vi "STD校准信息读取.vi"(8 "Error in":errorcluster caption="Error in (no error)", 11 "Slave ID":u8=1) -> (0 "error out":errorcluster, 2 "结果字符串":string, 3 "校准信息读取":T1 {"校准类型" items=["单点校准"=1, "两点校准"=2, "三点校准"=3]})   [LabVIEW 2016, in "斯坦道原位多参数.lvlib"]
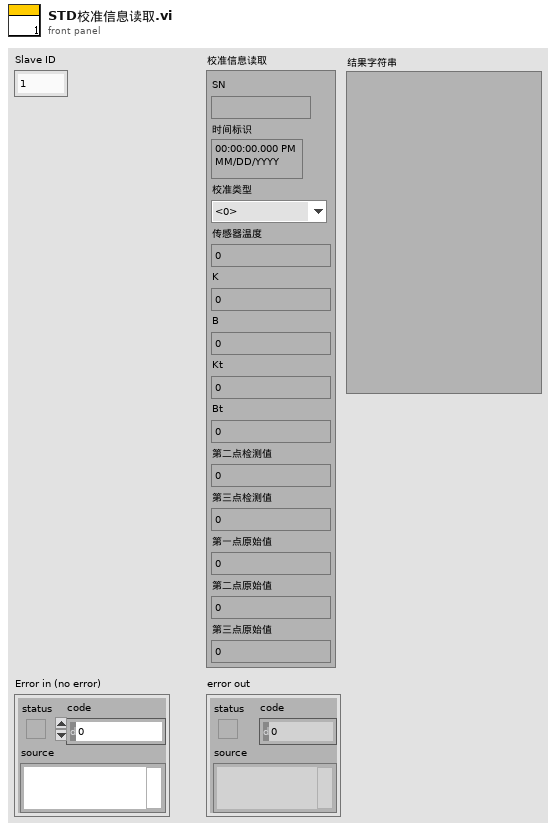
[diagram p1: front panel]
types:
  T1 = cluster{"SN":string, "时间标识":timestamp, "校准类型":u16, "传感器温度":sgl, "K":sgl, "B":sgl, "Kt":sgl, "Bt":sgl, "第二点检测值":sgl, "第三点检测值":sgl, "第一点原始值":sgl, "第二点原始值":sgl, "第三点原始值":sgl}
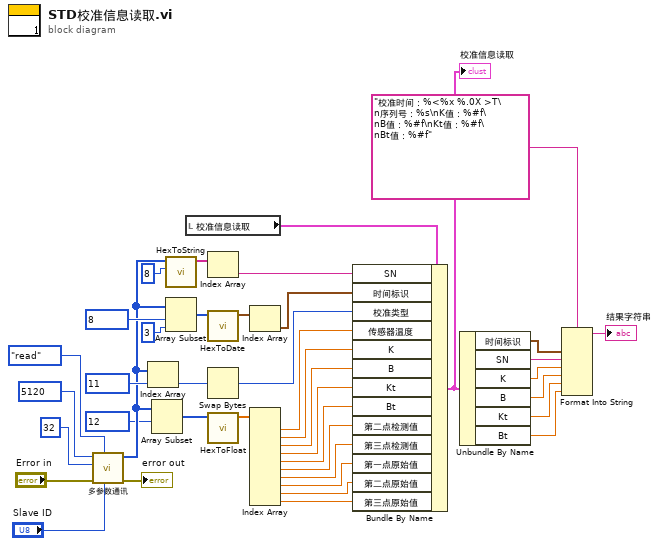
[diagram p0: block diagram]
diagram:
  n1 = call "多参数通讯.vi"("Slave ID"="Slave ID", "STEP"=enum16{"open", "read", "write", "close"}."read", "Error in"="Error in", "quantity"=u16 32, "starting address"=u16 5120) -> ("error out"=→"error out":errorcluster, "Registers"=w31:u16[])  [unwired: 4 in, 1 out]
  n2 = Index Array(array=w31, index=u16 11 ("starting address")) -> (element=w12:u16)
  n3 = Array Subset(array=w31, index=u16 12 ("starting address")) -> (w29:u16[])  [unwired: 1 in]
  n4 = call "HexToString.vi"("字符个数"=8, "数组"=w31) -> ("STRING"=w27:string[])  [unwired: 9 in]
  n5 = Array Subset(array=w31, index=u16 8 ("starting address"), length=3 ("长度")) -> (w33:u16[])
  n6 = local read "校准信息读取"() -> (w28:T1)
  n7 = Index Array(array=w27) -> (element=w26:string)  [unwired: 1 in]
  n8 = call "HexToDate.vi"("数组"=w33) -> ("DATE"=w25:timestamp[])  [unwired: 10 in]
  n9 = Swap Bytes(anything=w12) -> (byte swapped=w11:u16)
  n10 = call "HexToFloat.vi"("数组"=w29) -> ("FLOAT"=w23:sgl[])  [unwired: 10 in]
  n11 = Index Array(array=w25) -> (element=w24:timestamp)  [unwired: 1 in]
  n12 = Index Array(array=w23) -> (element #1=w22:sgl, element #2=w21:sgl, element #3=w20:sgl, element #4=w19:sgl, element #5=w18:sgl, element #6=w17:sgl, element #7=w16:sgl, element #8=w15:sgl, element #9=w14:sgl, element #10=w13:sgl)  [unwired: 10 in]
  n13 = Bundle By Name(cluster=w28, "SN"=w26, "时间标识"=w24, "校准类型"=w11, "传感器温度"=w22, "K"=w21, "B"=w20, "Kt"=w19, "Bt"=w18, "第二点检测值"=w17, "第三点检测值"=w16, "第一点原始值"=w15, "第二点原始值"=w14, "第三点原始值"=w13) -> (w8:T1)
  "校准信息读取" <- w8
  n14 = Unbundle By Name(w8) -> ("时间标识"=w7:timestamp, "SN"=w6:string, "K"=w5:sgl, "B"=w4:sgl, "Kt"=w3:sgl, "Bt"=w2:sgl)
  n15 = Format Into String(format string="校准时间：%<%x %.0X >T\n序列号：%s\nK值：%#f\nB值：%#f\nKt值：%#f\nBt值：%#f" ("格式字符串"), w7, w6, w5, w4, w3, w2) -> (resulting string=→"结果字符串":string)  [unwired: 2 in, 1 out]
